vi "Global_VALVE.vi"() -> ()   [LabVIEW 2015]
panel:
  out "Valve position OUT":u8
  out "VALVE ready":bool
  out "VALVE done":bool
  out "VALVE start":bool
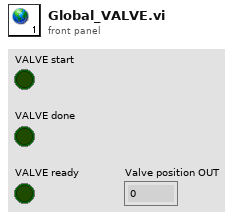
[diagram p1: front panel]
diagram:
